vi "RegisterTimer.vi"(6 "Start Imidiatlely?(F)":bool, 8 "error in (no error)":errorcluster, 9 "TimePeroid(ms)":i64, 10 "Name":string, 11 "UserEventTimer in":refnum<class "TimerEngine.lvclass">) -> (0 "error out":errorcluster, 2 "UserEvent":T1, 3 "UserEventTimer out":refnum<class "TimerEngine.lvclass">)   [LabVIEW 2017, in "TimerEngine.lvlib" / "TimerEngine.lvclass"]
uses:
  TimerEngine.lvclass
  _Typedef/Timer-UserEvent.ctl
  TimerEngine.lvclass/TimerEngine.ctl
  _TimerClass/Timer.lvclass/Timer.ctl
  _TimerClass/Timer.lvclass
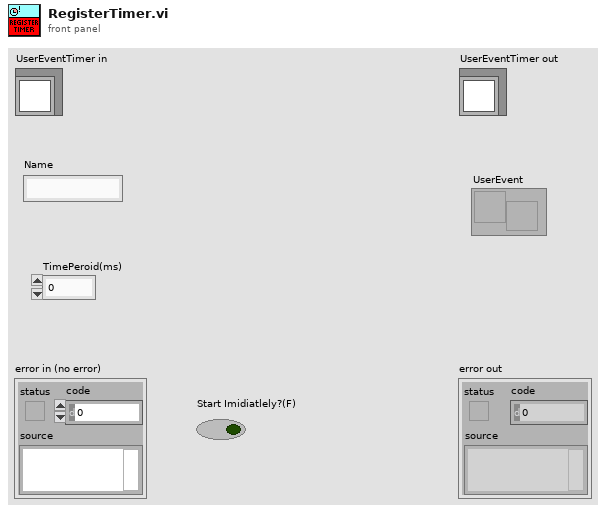
[diagram p1: front panel]
types:
  T1 = typedef "TimerEngine.lvlib/TimerEngine.lvclass/Timer-Userevent.ctl" = refnum<user-event>
  T2 = typedef "TimerEngine.lvlib/TimerEngine.lvclass/Timer-UserEvent.ctl" = refnum<user-event>
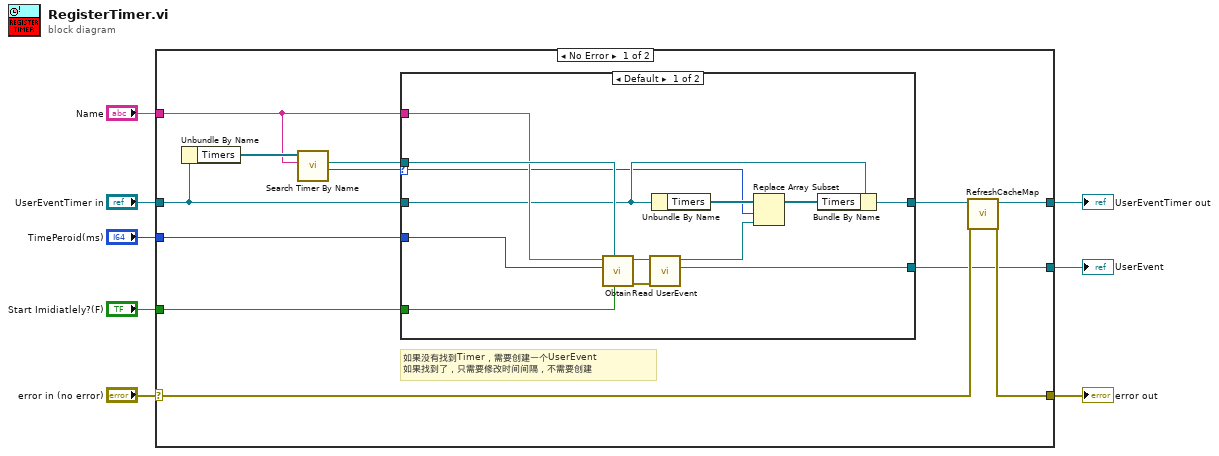
[diagram p0: block diagram]
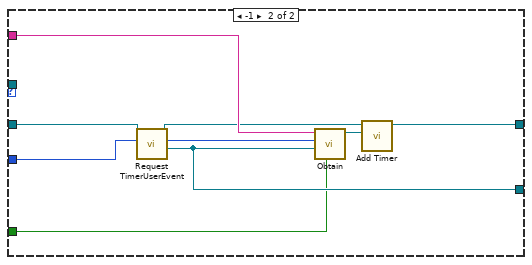
[diagram p2: hidden frame]
diagram:
  n1 = case shown="No Error" "error in (no error)" {
    selector: "error in (no error)" -> [w17 w44]
    tunnel: [w18 w44] -> w7
    tunnel: [w19 w43] -> w5
    tunnel: "UserEventTimer in" -> [w15 w43]
    tunnel: "Name" -> [w12 _]
    tunnel: "TimePeroid(ms)" -> [w20 _]
    tunnel: [w16 _] -> w2
    tunnel: "Start Imidiatlely?(F)" -> [w9 _]
    frame No Error {
      # "如果没有找到Timer，需要创建一个UserEvent\n如果找到了，只需要修改时间间隔，不需要创建"
      n2 = Unbundle By Name(w15) -> ("Timers"=w14:refnum<class "Timer.lvclass">[])
      n3 = call "Search Timer By Name.vi"("Name"=w12, "Array"=w14) -> ("index of element"=w13:i32, "element"=w10:refnum<class "Timer.lvclass">)  [unwired: 6 in, 2 out]
      n4 = case shown="Default" w13 {
        selector: w13 -> [w22 _]
        tunnel: w20 -> [w31 w42]
        tunnel: [w28 w40] -> w16
        tunnel: w15 -> [w26 w41]
        tunnel: w12 -> [w32 w38]
        tunnel: [w25 w35] -> w11
        tunnel: w10 -> [w33 _]
        tunnel: w9 -> [w21 w34]
        frame Default {
          n5 = call "Obtain.vi"("Start?"=w21, "Timer in"=w33, "TimePeroid(ms)"=w31, "Name"=w32) -> ("error out"=w29:errorcluster, "Timer out"=w30:refnum<class "Timer.lvclass">)  [unwired: 6 in]
          n6 = call "Read UserEvent.vi"("error in (no error)"=w29, "Timer in"=w30) -> ("UserEvent"=w28:T2, "Timer out"=w23:refnum<class "Timer.lvclass">)  [unwired: 7 in, 1 out]
          n7 = Unbundle By Name(w26) -> ("Timers"=w27:refnum<class "Timer.lvclass">[])
          n8 = Replace Array Subset(array=w27, new element=w23, index=w22) -> (w24:refnum<class "Timer.lvclass">[])
          n9 = Bundle By Name(cluster=w26, "Timers"=w24) -> (w25:refnum<class "TimerEngine.lvclass">)
        }
        frame -1 {
          n10 = call "Request TimerUserEvent.vi"("TimePeroid(ms)"=w42, "TimerEngine in"=w41) -> ("TimerUserEvent"=w40:T2, "TimePeroid(ms) OUT"=w39:i64, "TimerEngine out"=w37:refnum<class "TimerEngine.lvclass">)  [unwired: 6 in, 1 out]
          n11 = call "Obtain.vi"("Start?"=w34, "UserEvent"=w40, "TimePeroid(ms)"=w39, "Name"=w38) -> ("Timer out"=w36:refnum<class "Timer.lvclass">)  [unwired: 6 in, 1 out]
          n12 = call "Add Timer.vi"("Timer"=w36, "UserEventTimer in"=w37) -> ("UserEventTimer out"=w35:refnum<class "TimerEngine.lvclass">)  [unwired: 9 in]
        }
      }
      n13 = call "RefreshCacheMap.vi"("error in (no error)"=w17, "UserEventTimer in"=w11) -> ("error out"=w18:errorcluster, "UserEventTimer out"=w19:refnum<class "TimerEngine.lvclass">)  [unwired: 8 in]
    }
    frame Error {
    }
  }
  "error out" <- w7
  "UserEventTimer out" <- w5
  "UserEvent" <- w2
